vi "Build Transfer Group.vi"(8 "error in (no error)":errorcluster, 9 "inline?":bool, 10 "Transfer Group in":refnum<class "Transfer Group.lvclass">, 11 "Plugin Thread in":refnum<class "Plugin Thread.lvclass">) -> (0 "error out":errorcluster, 2 "Transfer Group out":refnum<class "Transfer Group.lvclass">, 3 "Plugin Thread out":refnum<class "Plugin Thread.lvclass">)   [LabVIEW 2017, in "DSF Core.lvlib" / "Plugin Thread.lvclass"]
uses:
  Plugin Thread.lvclass
  Transfer Group/Transfer Group.lvclass
  Plugin Thread.lvclass/Plugin Thread.ctl
  Buffer Converter/Buffer Converter.lvclass
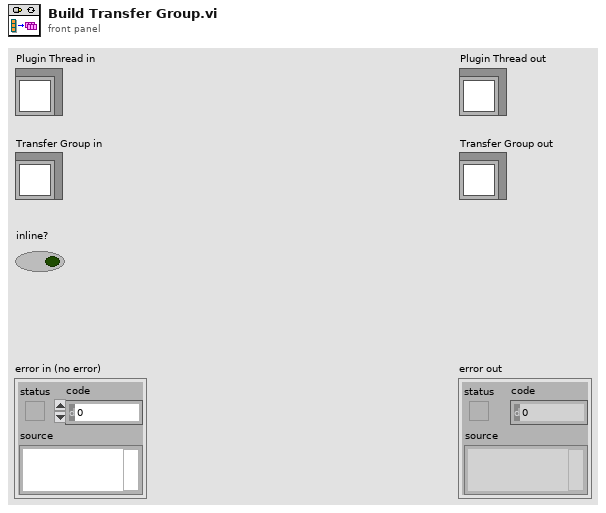
[diagram p1: front panel]
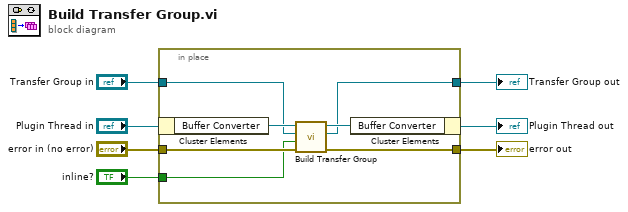
[diagram p0: block diagram]
diagram:
  n1 = in-place {
    in-place-border: "error in (no error)" -> [w12]
    in-place-border: [w11] -> w5
    in-place-border: "Transfer Group in" -> [w10]
    in-place-border: [w9] -> w2
    in-place-border: "inline?" -> [w8]
    n2 = in-place-cluster #1("Plugin Thread in") -> ("Buffer Converter"=w14:refnum<class "Buffer Converter.lvclass">)
    n3 = call "Build Transfer Group.vi"("error in (no error)"=w12, "inline?"=w8, "Transfer Group in"=w10, "Buffer Converter in"=w14) -> ("error out"=w11:errorcluster, "Transfer Group out"=w9:refnum<class "Transfer Group.lvclass">, "Buffer Converter out"=w13:refnum<class "Buffer Converter.lvclass">)  [unwired: 5 in]
    n4 = in-place-cluster #1("Buffer Converter"=w13) -> (→"Plugin Thread out":refnum<class "Plugin Thread.lvclass">)
  }
  "error out" <- w5
  "Transfer Group out" <- w2
